vi "AcqStart.vi"(6 "Delay between send and receive [ms]":i32=100, 8 "error in (no error)":errorcluster, 11 "SCD in":refnum<class "SCD.lvclass">) -> (0 "error out":errorcluster, 3 "SCD out":refnum<class "SCD.lvclass">)   [LabVIEW 2023, in "horiba.lvlib" / "SCD.lvclass"]
doc: "Define acquisition sets before starting an acquisition. Ensure acquisition preparation is completed successfully.\nStarting an acquisition will return an error if:\n\nAn acquisition is already running, or\nAcquisition preparation has not been completed.\nIn the event of errors in the defined parameters, the result will include an error_count field indicating the number of errors detected.\nuse saq3_getErrorLog to get the detailed error.\n\nTrigger Modes:\n\nMode description\n1 - 1st data started on Start command, all subsequent data acquired based on interval time\n2 - 1st data started by Trigger after start Command, all subsequent data acquired based on interval time\n3 - Each data acquisition waits for Trigger"
uses:
  SCD.lvclass
  SCD.lvclass/SCD.ctl
  b6349250-cb33-415b-847a-a7f5d99734f6.vi
  GenericDevice/GenericDevice.lvclass
  ca73f763-8e2b-4d84-8e4e-0e6044455bd1.vi
panel:
  in  "trigger":i32=1
  # "Connector Pane"
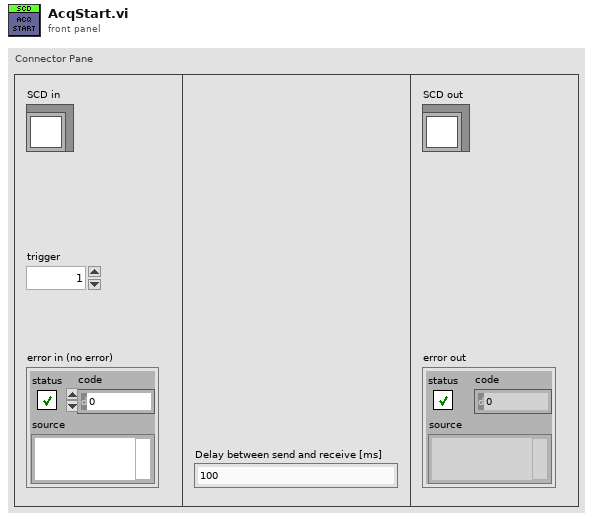
[diagram p1: front panel]
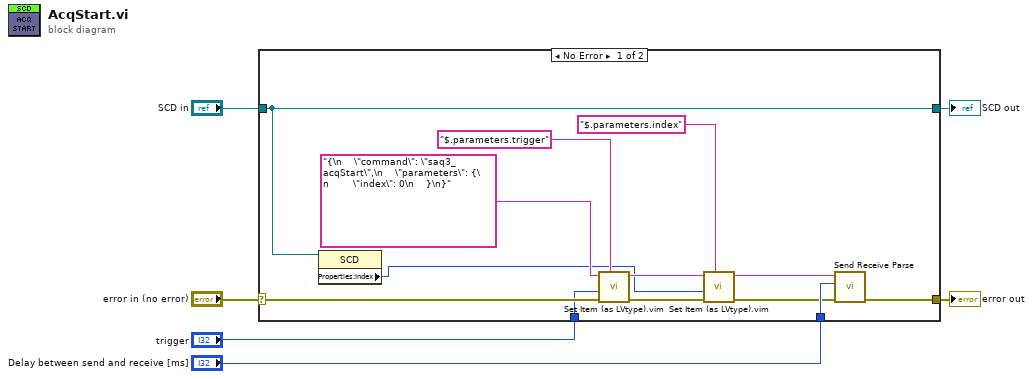
[diagram p0: block diagram]
diagram:
  n1 = case shown="No Error" "error in (no error)" {
    selector: "error in (no error)" -> [w17 w21]
    tunnel: [w15 w21] -> w2
    tunnel: [w18 w20] -> w4
    tunnel: "SCD in" -> [w18 w20]
    tunnel: "Delay between send and receive [ms]" -> [w14 _]
    tunnel: "trigger" -> [w10 _]
    frame No Error {
      n2 = property class="SCD"(reference=w18) -> ("Properties:Index"=w7:i32)  [unwired: 1 in, 2 out]
      n3 = call "Set Item (as LVtype).vim"("$Path or Item Name"="$.parameters.trigger", "error in (no error)"=w17, "Anything"=w10, "JSON"="{\n    \"command\": \"saq3_acqStart\",\n    \"parameters\": {\n        \"index\": 0\n    }\n}") -> ("error out"=w16:errorcluster, "<JSON>"=w12:string)  [unwired: 4 in, 1 out]
      n4 = call "Set Item (as LVtype).vim"("$Path or Item Name"="$.parameters.index", "error in (no error)"=w16, "Anything"=w7, "JSON"=w12) -> ("error out"=w13:errorcluster, "<JSON>"=w11:string)  [unwired: 4 in, 1 out]
      n5 = call "Send Receive Parse.vi"("error in"=w13, "Delay between send and receive [ms]"=w14, "<JSON>"=w11) -> ("error out"=w15:errorcluster)  [unwired: 6 in, 2 out]
    }
    frame Error {
    }
  }
  "error out" <- w2
  "SCD out" <- w4
